vi "Get Property.vi"(10 "Ctl Ref":refnum<vi>, 11 "UIP In":refnum<class "SizeUIP.lvclass">) -> (0 "Error Out":errorcluster, 3 "UIP Out":refnum<class "SizeUIP.lvclass">)   [LabVIEW 2015, in "SizeUIP.lvclass"]
doc: "Modify this method to implement functionality for extracting the property from VI Server Control to be stored inside UIP."
uses:
  SizeUIP.lvclass
  SizeUIP.lvclass/SizeUIP.ctl
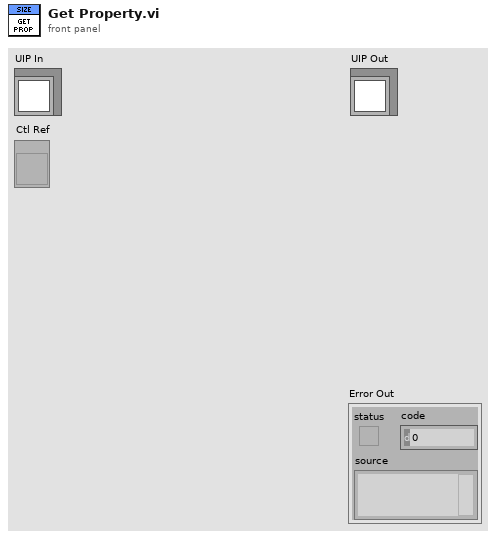
[diagram p1: front panel]
types:
  T1 = typedef "LVBoundsTypeDef.ctl" = cluster{"Width":u32, "Height":u32}
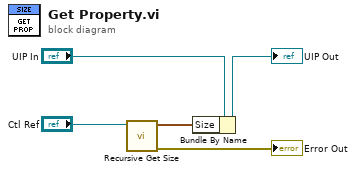
[diagram p0: block diagram]
diagram:
  n1 = call "Recursive Get Size.vi"("Control"="Ctl Ref") -> ("error out"=→"Error Out":errorcluster, "Size"=w2:T1)  [unwired: 9 in]
  n2 = Bundle By Name(cluster="UIP In", "Size"=w2) -> (→"UIP Out":refnum<class "SizeUIP.lvclass">)
